vi "Colimation Steps.vi"(0 "Motion Controller in":refnum<class "Motion Controller.lvclass">, 1 "Steps":dbl[unit][](array[numeric]), 2 "Cancel?":bool, 5 "Beam Profiler in":refnum<class "Beam Profiler.lvclass">, 7 "Peak responsivity [%,0-100]":dbl, 9 "Knife Edge in":T1={"X"=nan, "Y"=nan}, 11 "Error in":errorcluster, 12 "Start Position":dbl[unit], 13 "Stop Collimation Position":dbl[unit]) -> (3 "Cancel Test":bool, 4 "Motion Controller out":refnum<class "Motion Controller.lvclass">, 6 "Beam Profiler out":refnum<class "Beam Profiler.lvclass">, 8 "Stop Position":dbl[unit], 14 "Steps data":dbl[][](array[numeric]), 15 "Error out":errorcluster)   [LabVIEW 2018]
uses:
  <instrlib>/nLight Instruments/Motion Controller/Motion Controller.lvclass
  <instrlib>/nLight Instruments/Beam Profiler/Beam profiler XY distance value pair.ctl
  <instrlib>/nLight Instruments/Beam Profiler/Beam Profiler.lvclass
  <instrlib>/nLight Instruments/Motion Controller/Axis index.ctl
  <instrlib>/nLight Instruments/Motion Controller/Move axis absolute distance units.vi
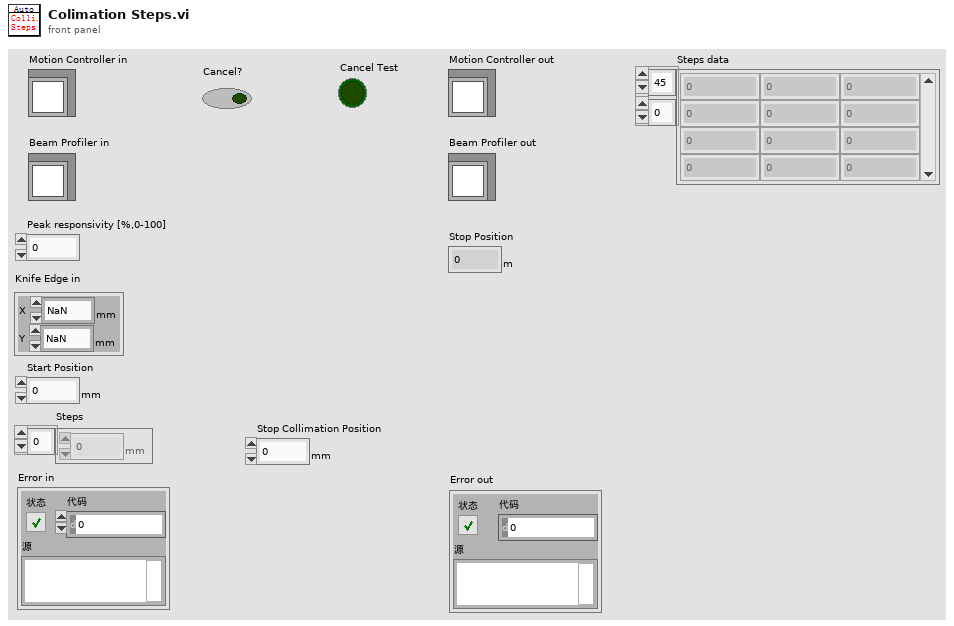
[diagram p1: front panel]
types:
  T1 = typedef "Beam Profiler.lvclass/Beam profiler XY distance value pair.ctl" = cluster{"X":dbl[unit], "Y":dbl[unit]}
  T2 = typedef "Motion Controller.lvclass/Axis index.ctl" = i32
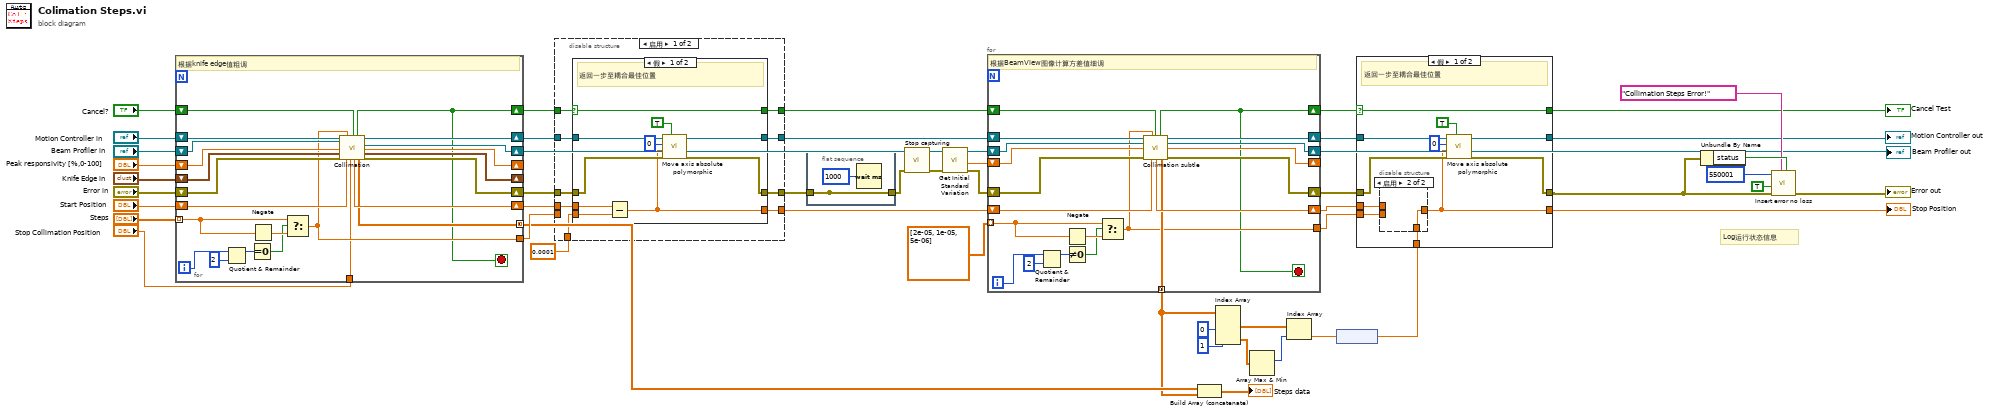
[diagram p0: block diagram]
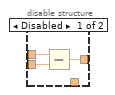
[diagram p4: hidden frame]
diagram:
  # "Log运行状态信息"
  n1 = for {
    shift-right: [w54] -> w37
    shift-left: "Cancel?" -> [w69]
    shift-right: [w68] -> w45
    shift-left: "Motion Controller in" -> [w75]
    shift-right: [w67] -> w12
    shift-left: "Beam Profiler in" -> [w74]
    shift-right: [w66] -> _
    shift-left: "Peak responsivity [%,0-100]" -> [w73]
    shift-right: [w65] -> _
    shift-left: "Knife Edge in" -> [w72]
    shift-right: [w57] -> w44
    shift-left: "Error in" -> [w71]
    shift-right: [w64] -> w43
    shift-left: "Start Position" -> [w70]
    tunnel: "Steps" -> [w59] mode=indexing
    tunnel: [w56] -> w27 mode=concatenating
    tunnel: [w55] -> w42
    tunnel: "Stop Collimation Position" -> [w53]
    i -> [w58]
    stop <- w54 stop-if-true
    # "根据knife edge值粗调"
    n2 = Quotient & Remainder(x=w58, y=2) -> (x-y*floor(x/y)=w60:i32)  [unwired: 1 out]
    n3 = Equal To 0?(x=w60) -> (x = 0?=w61:bool)
    n4 = Negate(x=w59) -> (-x=w63:dbl[unit])
    n5 = Select(t=w59, s=w61, f=w63) -> (s? t:f=w55:dbl[unit])
    n6 = call "Collimation.vi"("Motion Controller in"=w75, "Beam Profiler in"=w74, "Peak responsivity [%,0-100]"=w73, "Knife Edge in"=w72, "Error in"=w71, "Step"=w55, "Start Position"=w70, "Stop Collimation Position"=w53, "Cancel?"=w69) -> ("Stop positon"=w64:dbl[unit], "Cancel Test"=w54:bool, "数组"=w56:dbl[][], "Motion Controller out"=w68:refnum<class "Motion Controller.lvclass">, "Beam Profiler out"=w67:refnum<class "Beam Profiler.lvclass">, "Peak responsivity [%,0-100] out"=w66:dbl, "Knife Edge out"=w65:T1, "Error out"=w57:errorcluster)  [unwired: 3 in]
  }
  n7 = disable-structure shown="启用" {
    disable-tunnel: w45 -> [w84 w101]
    disable-tunnel: w44 -> [w83 w100]
    disable-tunnel: w43 -> [w82 w99]
    disable-tunnel: w42 -> [_ _]
    disable-tunnel: w37 -> [w81 w102]
    disable-tunnel: [w80 w102] -> w36
    disable-tunnel: [w79 w101] -> w35
    disable-tunnel: [w78 w99] -> w34
    disable-tunnel: [w77 w100] -> w2
    disable-tunnel: dbl[unit] 0.0001 ("Step") -> [w76 _]
    frame Enabled {
      n8 = case shown="假" w81 {
        selector: w81 -> [w86 w96]
        tunnel: w84 -> [w92 w98]
        tunnel: w83 -> [w91 w97]
        tunnel: w82 -> [w88 w95]
        tunnel: [w90 w98] -> w79
        tunnel: [w89 w97] -> w77
        tunnel: w76 -> [w87 _]
        tunnel: [w86 w96] -> w80
        tunnel: [w85 w95] -> w78
        frame False {
          # "返回一步至耦合最佳位置"
          n9 = Subtract(x=w88, y=w87) -> (x-y=w85:dbl[unit])
          n10 = call-poly <instrlib>:"Move axis absolute polymorphic.vi"("Wait? (T)"=TRUE, "error in (no error)"=w91, "Move location"=w85, "Axis index"=T2 0, "Motion Controller in"=w92) -> ("error out"=w89:errorcluster, "Motion Controller out"=w90:refnum<class "Motion Controller.lvclass">)  [unwired: 5 in]
        }
        frame True {
        }
      }
    }
    frame Disabled {
    }
  }
  n11 = flat-sequence {
    tunnel: w2 -> [w103]
    tunnel: [w103] -> _
    tunnel: [w103] -> w1
    frame #0 {
      n12 = Wait (ms)(milliseconds to wait=u32 1000 ("等待时间（毫秒）")) -> ()  [unwired: 1 out]
    }
  }
  n13 = call-dynamic "Stop capturing.vi"("error in (no error)"=w1, "Beam Profiler in"=w12) -> ("error out"=w13:errorcluster, "Beam Profiler out"=w11:refnum<class "Beam Profiler.lvclass">)  [unwired: 8 in]
  n14 = call "Get Initial Standard Variation.vi"("Error in"=w13, "Beam Profiler in"=w11) -> ("Error out"=w29:errorcluster, "Standard Variation"=w30:sgl, "Beam Profiler out"=w31:refnum<class "Beam Profiler.lvclass">)  [unwired: 7 in]
  n15 = for {
    shift-right: [w105] -> w26
    shift-left: w36 -> [w118]
    shift-right: [w121] -> w22
    shift-left: w29 -> [w122]
    shift-right: [w120] -> w15
    shift-left: w31 -> [w123]
    shift-right: [w119] -> w24
    shift-left: w35 -> [w124]
    tunnel: dbl[unit][] [2e-05, 1e-05, 5e-06] ("Steps") -> [w111] mode=indexing
    shift-right: [w116] -> w20
    shift-left: w34 -> [w117]
    shift-right: [w108] -> _
    shift-left: w30 -> [w109]
    tunnel: [w107] -> w10 mode=concatenating
    tunnel: [w106] -> w19
    i -> [w110]
    stop <- w105 stop-if-true
    # "根据BeamView图像计算方差值细调"
    n16 = Quotient & Remainder(x=w110, y=2) -> (x-y*floor(x/y)=w112:i32)  [unwired: 1 out]
    n17 = Not Equal To 0?(x=w112) -> (x != 0?=w113:bool)
    n18 = Negate(x=w111) -> (-x=w115:dbl[unit])
    n19 = Select(t=w111, s=w113, f=w115) -> (s? t:f=w106:dbl[unit])
    n20 = call "Collimation subtle.vi"("Motion Controller in"=w124, "Step"=w106, "Cancel?"=w118, "Beam Profiler in"=w123, "Standard Variation in"=w109, "Error in"=w122, "Start Position"=w117) -> ("Cancel Test"=w105:bool, "Motion Controller out"=w119:refnum<class "Motion Controller.lvclass">, "Beam Profiler out"=w120:refnum<class "Beam Profiler.lvclass">, "Standard Variation out"=w108:dbl, "Stop positon"=w116:dbl[unit], "subtle data"=w107:dbl[][], "Error out"=w121:errorcluster)  [unwired: 2 in]
  }
  "Beam Profiler out" <- w15
  n21 = Build Array (concatenate)(w27, w10) -> (→"Steps data":dbl[][])
  n22 = Index Array(array=w10, index (col) #1=0 ("禁用的索引 (列)"), index (col) #2=1 ("索引 (列)")) -> (element #1=w6:dbl[], element #2=w7:dbl[])  [unwired: 2 in]
  n23 = Array Max & Min(array=w7) -> (max index (indices)=w5:i32)  [unwired: 3 out]
  n24 = Index Array(array=w6, index=w5) -> (element=w4:dbl)
  n25 = node(w4) -> (w3:dbl[unit])
  n26 = case shown="假" w26 {
    selector: w26 -> [w127 w141]
    tunnel: w24 -> [w133 w143]
    tunnel: w22 -> [w132 w142]
    tunnel: w20 -> [w129 w140]
    tunnel: [w131 w143] -> w23
    tunnel: [w130 w142] -> w21
    tunnel: w19 -> [w128 _]
    tunnel: [w127 w141] -> w25
    tunnel: [w126 w140] -> w18
    tunnel: w3 -> [w125 _]
    frame False {
      # "返回一步至耦合最佳位置"
      n27 = disable-structure shown="启用" {
        disable-tunnel: w129 -> [w138 _]
        disable-tunnel: w128 -> [w137 _]
        disable-tunnel: [w136 w139] -> w126
        disable-tunnel: w125 -> [_ w139]
        frame Disabled {
          n28 = Subtract(x=w138, y=w137) -> (x-y=w136:dbl[unit])
        }
        frame Enabled {
        }
      }
      n29 = call-poly <instrlib>:"Move axis absolute polymorphic.vi"("Wait? (T)"=TRUE, "error in (no error)"=w132, "Move location"=w126, "Axis index"=T2 0, "Motion Controller in"=w133) -> ("error out"=w130:errorcluster, "Motion Controller out"=w131:refnum<class "Motion Controller.lvclass">)  [unwired: 5 in]
    }
    frame True {
    }
  }
  "Motion Controller out" <- w23
  "Cancel Test" <- w25
  "Stop Position" <- w18
  n30 = Unbundle By Name(w21) -> ("status"=w40:bool)
  n31 = call <userlib>:"Insert error no loss.vi"("Add error? (T)"=w40, "error message"="Collimation Steps Error!" ("format string"), "error in (no error)"=w21, "Error = T, Warning = F (T)"=TRUE, "error code"=550001) -> ("error out"=→"Error out":errorcluster)  [unwired: 4 in]
